vi "Check first message.vi"(8 "error in (no error)":errorcluster, 9 "First Message":string, 10 "Remote Address":string, 11 "TCP Listener in":refnum<class "TCP Listener.lvclass">) -> (0 "error out":errorcluster, 3 "TCP Listener out":refnum<class "TCP Listener.lvclass">)   [LabVIEW 2026, in "TALOS.lvlib" / "TCP Listener.lvlib" / "TCP Listener.lvclass"]
uses:
  TCP Listener.lvclass
  Ancestor/Ancestor/Ancestor.lvclass/Ancestor.ctl
  Support VIs/Circus Config Param - Core.vi
  FGV/Error Memory/Get Error Description.vi
  Ancestor/Ancestor/Read ID.vi
  Support VIs/Get Class Name.vi
  <vilib>/Utility/error.llb/Clear Errors.vi
  Support VIs/Circus Root Path.vi
  Support VIs/TALOS Config Param.vi
  FGV/Error Memory/Error Memory Core.vi
  <vilib>/AdvancedString/Delimited String to 1D String Array.vi
  <vilib>/AdvancedString/Delimited String to 1D String Array (string).vi
  FGV/Error Memory/Error Crt Lvl checker.vi
  FGV/Error Memory/Error Memory Core.vi/40c8088d-b597-4017-91af-faa98e00292e.vi
  FGV/Error Memory/Error Memory Core.vi/d4a3ab98-063c-4e44-b43d-fbdcfe6c2be2.vi
  Support VIs/Global Memory.vi
  <vilib>/Utility/LVClass/Get LV Class Name.vi
  Support VIs/Is in Packed Library.vi
  Support VIs/TALOS Root path.vi
  Support VIs/Read CSV worksheet.vi
  Support VIs/Global Constants.vi
  <vilib>/Utility/error.llb/General Error Handler.vi
  <vilib>/Utility/config.llb/Open Config Data.vi
  <vilib>/Utility/config.llb/Get Section Names.vi
  <vilib>/Utility/config.llb/Get Key Names.vi
  <vilib>/Utility/config.llb/Read Key.vi
  <vilib>/Utility/config.llb/Read Key (String).vi
  <vilib>/Utility/config.llb/Close Config Data.vi
  Guardian/Guardian/Extract list from Project INI file entry.vi
  Ancestor/Ancestor/Ancestor.lvclass
  <vilib>/Comparison/Equal/Equal Functor/Equal Functor.lvclass
  TALOS.lvlib
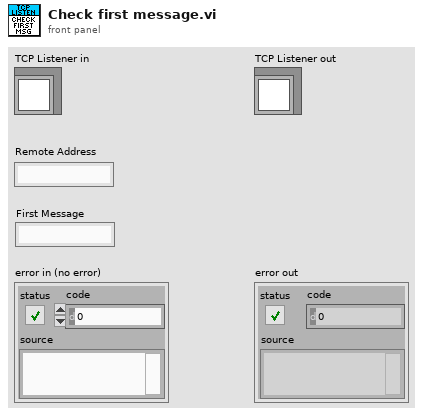
[diagram p1: front panel]
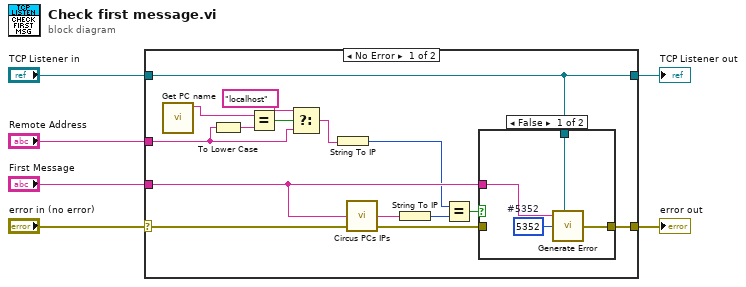
[diagram p0: block diagram]
diagram:
  n1 = case shown="No Error" "error in (no error)" {
    selector: "error in (no error)" -> [w21 w27]
    tunnel: "First Message" -> [w16 _]
    tunnel: "Remote Address" -> [w8 _]
    tunnel: [w18 w27] -> w3
    tunnel: [w17 w28] -> w2
    tunnel: "TCP Listener in" -> [w17 w28]
    frame No Error {
      n2 = call "Get PC name.vi"() -> ("Hostname"=w12:string)  [unwired: 10 in, 1 out]
      n3 = To Lower Case(string=w8) -> (all lower case string=w11:string)
      n4 = Equal?(x=w12, y=w11) -> (x = y?=w10:bool)
      n5 = Select(t="localhost", s=w10, f=w8) -> (s? t:f=w9:string)
      n6 = String To IP(1:w9) -> (0:w13:u32)
      n7 = call "Circus PCs IPs.vi"("error in (no error)"=w21, "ID"=w16) -> ("error out"=w19:errorcluster, "IP"=w15:string)  [unwired: 2 in]
      n8 = String To IP(1:w15) -> (0:w14:u32)
      n9 = Equal?(x=w13, y=w14) -> (x = y?=w20:bool)
      n10 = case shown="False" w20 {
        tunnel: w19 -> [_ w26]
        tunnel: [w25 w26] -> w18
        tunnel: w17 -> [w24 _]
        tunnel: w16 -> [w23 _]
        frame False {
          w22 = 5352  # #5352
          n11 = call "Generate Error.vi"("Optional String"=w23, "Class"=w24, "Error Code"=w22) -> ("error out"=w25:errorcluster)  [unwired: 4 in]
        }
        frame True {
        }
      }
    }
    frame Error {
    }
  }
  "error out" <- w3
  "TCP Listener out" <- w2
